vi "aggregator - ii - real.vi"(0 "number":dbl, 1 "requested size":i32=20, 3 "requested averaging interval":i32=10, 12 "first time":bool) -> (4 "Array":dbl[](array[numeric]), 6 "interp array":dbl[](array[numeric]), 10 "mean array":dbl[](array[numeric]), 13 "intercept":dbl, 14 "slope":dbl, 15 "interpolated average":dbl)   [LabVIEW 2015]
panel:
  out "actual number of elements":i32
  out "mean":dbl
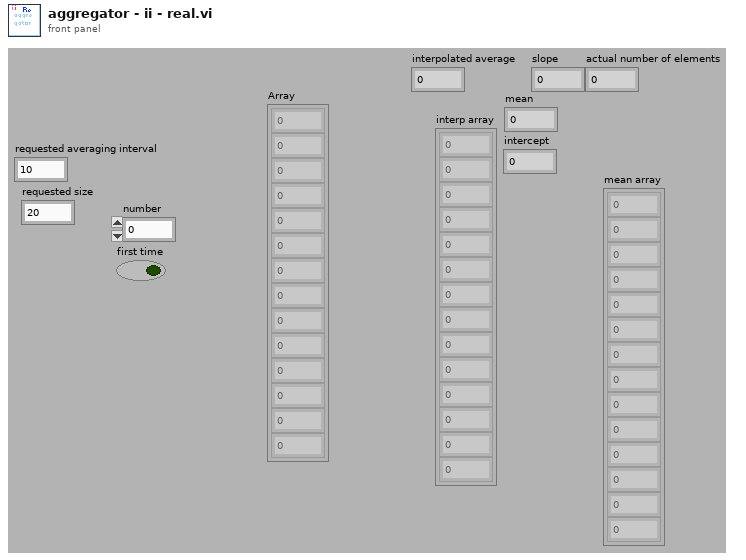
[diagram p1: front panel]
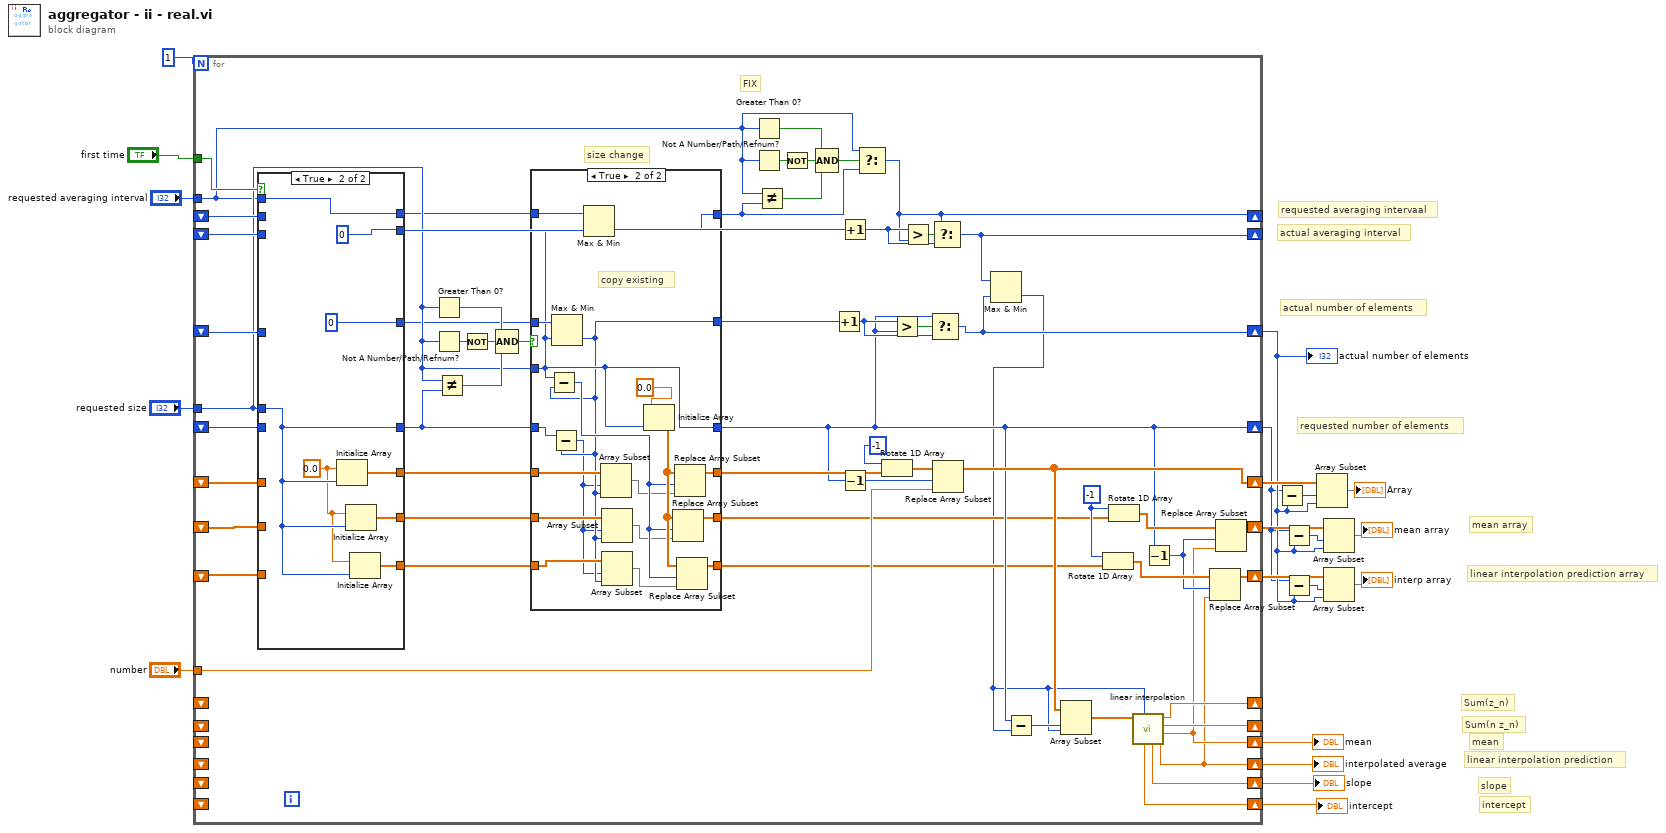
[diagram p0: block diagram]
diagram:
  # "actual averaging interval"
  # "requested averaging intervaal"
  # "linear interpolation prediction"
  # "mean"
  # "intercept"
  # "slope"
  # "linear interpolation prediction array"
  # "mean array"
  # "Sum(n z_n)"
  # "Sum(z_n)"
  # "requested number of elements"
  # "actual number of elements"
  n1 = for {
    N: 1 -> [_]
    tunnel: "first time" -> [w56]
    shift-right: [w24] -> w6
    shift-left: _ -> [w80]
    tunnel: "requested size" -> [w42]
    tunnel: "number" -> [w75]
    shift-right: [w58] -> w16
    shift-left: _ -> [w77]
    shift-right: [w39] -> w5
    shift-left: _ -> [w72]
    shift-right: [w65] -> w10
    shift-left: _ -> [w71]
    shift-right: [w64] -> w7
    shift-left: _ -> [w70]
    shift-right: [w55] -> _
    shift-left: _ -> [_]
    shift-right: [w54] -> _
    shift-left: _ -> [_]
    shift-right: [w51] -> w3
    shift-left: _ -> [_]
    shift-right: [w50] -> w1
    shift-left: _ -> [_]
    shift-right: [w53] -> w2
    shift-left: _ -> [_]
    shift-right: [w52] -> w4
    shift-left: _ -> [_]
    shift-right: [w23] -> _
    shift-left: _ -> [w60]
    shift-right: [w25] -> _
    shift-left: _ -> [w59]
    tunnel: "requested averaging interval" -> [w27]
    w67 = -1 ("n")
    # "FIX"
    # "size change"
    n2 = case shown="True" w56 {
      tunnel: w80 -> [w111 _]
      tunnel: [w111 0] -> w40
      tunnel: w77 -> [w108 _]
      tunnel: w42 -> [_ w114]
      tunnel: w72 -> [w109 _]
      tunnel: w71 -> [w107 _]
      tunnel: w70 -> [w106 _]
      tunnel: [w108 w117] -> w44
      tunnel: [w107 w116] -> w36
      tunnel: [w106 w115] -> w37
      tunnel: [w112 0] -> w62
      tunnel: w60 -> [w112 _]
      tunnel: w27 -> [_ w118]
      tunnel: w59 -> [w110 _]
      tunnel: [w110 w118] -> w33
      tunnel: [w109 w114] -> w41
      frame False {
      }
      frame True {
        w113 = 0.0
        n3 = Initialize Array(w113, w114) -> (w117:dbl[])
        n4 = Initialize Array(w113, w114) -> (w116:dbl[])
        n5 = Initialize Array(w113, w114) -> (w115:dbl[])
      }
    }
    n6 = Greater Than 0?(x=w42) -> (x > 0?=w48:bool)
    n7 = Not A Number/Path/Refnum?(number/path/refnum=w42) -> (NaN/Path/Refnum?=w49:bool)
    n8 = Not Equal?(x=w42, y=w41) -> (x != y?=w46:bool)
    n9 = Not(x=w49) -> (.not. x?=w47:bool)
    n10 = Compound Arithmetic op=AND(w48, w47, w46) -> (w45:bool)
    n11 = case shown="True" w45 {
      tunnel: [w86 w88] -> w38
      tunnel: w40 -> [w86 w104]
      tunnel: [w85 w96] -> w39
      tunnel: w41 -> [w85 w89]
      tunnel: [w84 w103] -> w43
      tunnel: w44 -> [w84 w95]
      tunnel: w42 -> [_ w96]
      tunnel: w37 -> [w82 w93]
      tunnel: w36 -> [w83 w91]
      tunnel: [w83 w102] -> w35
      tunnel: [w82 w101] -> w34
      tunnel: w33 -> [w81 w98]
      tunnel: [w81 w97] -> w26
      frame False {
      }
      frame True {
        # "copy existing"
        n12 = Max & Min(x=w104, y=w96) -> (min(x,y)=w88:i32)  [unwired: 1 out]
        n13 = Subtract(x=w96, y=w88) -> (x-y=w99:i32)
        n14 = Subtract(x=w89, y=w88) -> (x-y=w87:i32)
        n15 = Max & Min(x=w98, y=w96) -> (min(x,y)=w97:i32)  [unwired: 1 out]
        n16 = Array Subset(array=w95, index=w87, length=w88) -> (w94:dbl[])
        n17 = Array Subset(array=w91, index=w87, length=w88) -> (w90:dbl[])
        n18 = Array Subset(array=w93, index=w87, length=w88) -> (w92:dbl[])
        n19 = Initialize Array(0.0, w96) -> (w100:dbl[])
        n20 = Replace Array Subset(array=w100, new element=w90, index=w99) -> (w102:dbl[])
        n21 = Replace Array Subset(array=w100, new element=w94, index=w99) -> (w103:dbl[])
        n22 = Replace Array Subset(array=w100, new element=w92, index=w99) -> (w101:dbl[])
      }
    }
    n23 = Greater Than 0?(x=w27) -> (x > 0?=w31:bool)
    n24 = Not A Number/Path/Refnum?(number/path/refnum=w27) -> (NaN/Path/Refnum?=w32:bool)
    n25 = Not Equal?(x=w27, y=w26) -> (x != y?=w29:bool)
    n26 = Not(x=w32) -> (.not. x?=w30:bool)
    n27 = Compound Arithmetic op=AND(w31, w30, w29) -> (w28:bool)
    n28 = Increment(x=w38) -> (x+1=w78:i32)
    n29 = Increment(x=w62) -> (x+1=w61:i32)
    n30 = Decrement(x=w39) -> (x-1=w74:i32)
    n31 = Select(t=w27, s=w28, f=w26) -> (s? t:f=w25:i32)
    n32 = Rotate 1D Array(1:w43, 2:-1 ("n")) -> (0:w73:dbl[])
    n33 = Greater?(x=w78, y=w39) -> (0:w79:bool)
    n34 = Greater?(x=w61, y=w25) -> (0:w63:bool)
    n35 = Select(t=w39, s=w79, f=w78) -> (s? t:f=w24:i32)
    n36 = Select(t=w25, s=w63, f=w61) -> (s? t:f=w23:i32)
    n37 = Replace Array Subset(array=w73, new element=w75, index=w74) -> (w58:dbl[])
    n38 = Max & Min(x=w23, y=w24) -> (min(x,y)=w22:i32)  [unwired: 1 out]
    n39 = Subtract(x=w39, y=w22) -> (x-y=w57:i32)
    n40 = Array Subset(array=w58, index=w57, length=w22) -> (w21:dbl[])
    n41 = Rotate 1D Array(1:w34, 2:w67) -> (0:w68:dbl[])
    n42 = Rotate 1D Array(1:w35, 2:w67) -> (0:w69:dbl[])
    n43 = call "linear interpolation.vi"("n"=w22, "Array"=w21) -> ("interpolated average"=w52:cdb, "mean"=w53:cdb, "sum n z_n"=w54:cdb, "sum z_n"=w55:cdb, "slope"=w51:cdb, "intercept"=w50:cdb)  [unwired: 4 in]
    n44 = Decrement(x=w39) -> (x-1=w66:i32)
    n45 = Replace Array Subset(array=w68, new element=w52, index=w66) -> (w64:dbl[])
    n46 = Replace Array Subset(array=w69, new element=w53, index=w66) -> (w65:dbl[])
  }
  "interpolated average" <- w4
  "slope" <- w3
  "mean" <- w2
  "actual number of elements" <- w6
  "intercept" <- w1
  n47 = Subtract(x=w5, y=w6) -> (x-y=w14:i32)
  n48 = Subtract(x=w5, y=w6) -> (x-y=w11:i32)
  n49 = Subtract(x=w5, y=w6) -> (x-y=w8:i32)
  n50 = Array Subset(array=w16, index=w14, length=w6) -> (→"Array":dbl[])
  n51 = Array Subset(array=w10, index=w11, length=w6) -> (→"mean array":dbl[])
  n52 = Array Subset(array=w7, index=w8, length=w6) -> (→"interp array":dbl[])
